vi "Fix Fixed-Point Configuration on Representation Change.vi"(8 "error in (no error)":errorcluster, 11 "Numeric Data Type in":refnum<class "Numeric Data Type.lvclass">) -> (0 "error out":errorcluster, 3 "Numeric Data Type out":refnum<class "Numeric Data Type.lvclass">)   [LabVIEW 2018, in "Numeric Data Type.lvclass"]
uses:
  Numeric Data Type.lvclass
  Fixed-Point Value.ctl
  Numeric Data Type.lvclass/Numeric Data Type.ctl
  <vilib>/fxp/FXPxcontrol/FXP.xctl
  Reference Fixed-Point Configuration.vi
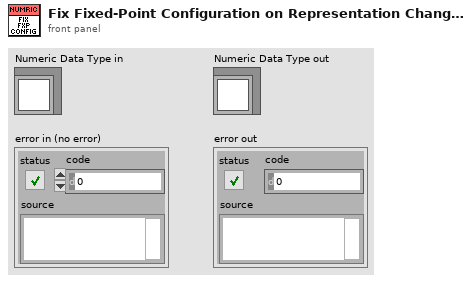
[diagram p1: front panel]
types:
  T1 = typedef "Numeric Data Type.lvclass/Fixed-Point Value.ctl" = cluster{"Encoding":cluster{"Signed":bool, "Word Length":u32, "Integer Word Length":i32}, "Range":cluster{"Range Min":dbl, "Range Max":dbl, "Delta":dbl}}
  T2 = typedef "Numeric Data Type.lvclass/Representation Enum.ctl" = enum16{"Extended (EXT)", "Double (DBL)", "Single (SGL)", "Fixed-Point (FXP)", "Quad Integer (I64)", "Long Integer (I32)", "Word Integer (I16)", "Byte Integer (I8)", "Unsigned Quad (U64)", "Unsigned Long (U32)", "Unsigned Word (U16)", "Unsigned Byte (U8)", "Complex Extended (CXT)", "Complex Double (CDB)", "Complex Single (CSG)"}
  T3 = enum8{"Enabled", "Disabled", "Disabled and Grayed Out"}
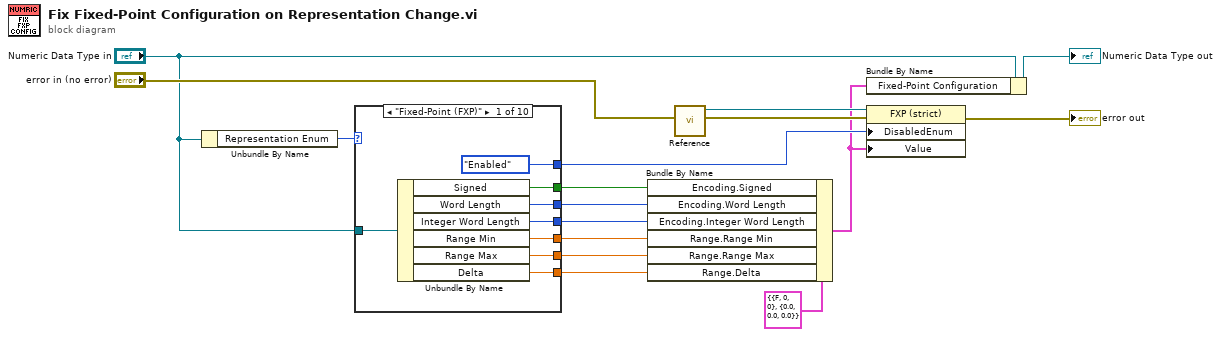
[diagram p0: block diagram]
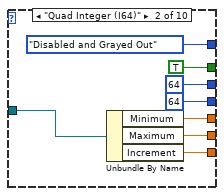
[diagram p2: hidden frame]
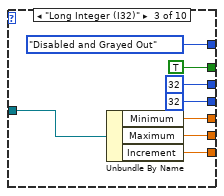
[diagram p3: hidden frame]
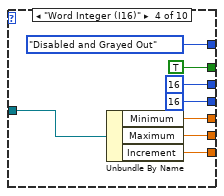
[diagram p4: hidden frame]
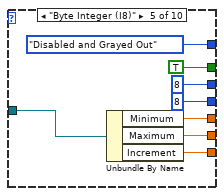
[diagram p5: hidden frame]
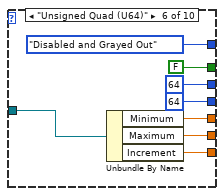
[diagram p6: hidden frame]
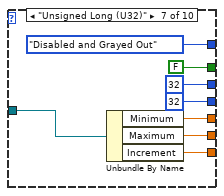
[diagram p7: hidden frame]
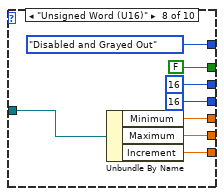
[diagram p8: hidden frame]
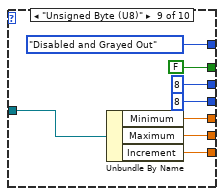
[diagram p9: hidden frame]
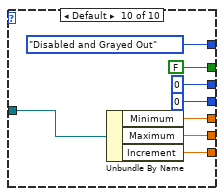
[diagram p10: hidden frame]
diagram:
  n1 = Unbundle By Name("Numeric Data Type in") -> ("Representation Enum"=w14:T2)
  n2 = case shown="\"Fixed-Point (FXP)\"" w14 {
    tunnel: [T3."Enabled" ("Disabled") T3."Disabled and Grayed Out" ("Disabled") T3."Disabled and Grayed Out" ("Disabled") T3."Disabled and Grayed Out" ("Disabled") T3."Disabled and Grayed Out" ("Disabled") T3."Disabled and Grayed Out" ("Disabled") T3."Disabled and Grayed Out" ("Disabled") T3."Disabled and Grayed Out" ("Disabled") T3."Disabled and Grayed Out" ("Disabled") T3."Disabled and Grayed Out" ("Disabled")] -> w7
    tunnel: "Numeric Data Type in" -> [w17 w28 w36 w44 w52 w60 w68 w76 w84 w92]
    tunnel: [w23 TRUE TRUE TRUE TRUE FALSE FALSE FALSE FALSE FALSE] -> w8
    tunnel: [w22 u32 64 u32 32 u32 16 u32 8 u32 64 u32 32 u32 16 u32 8 u32 0] -> w9
    tunnel: [w21 64 32 16 8 64 32 16 8 0] -> w10
    tunnel: [w20 w27 w35 w43 w51 w59 w67 w75 w83 w91] -> w11
    tunnel: [w19 w26 w34 w42 w50 w58 w66 w74 w82 w90] -> w12
    tunnel: [w18 w25 w33 w41 w49 w57 w65 w73 w81 w89] -> w13
    frame "Fixed-Point (FXP)" {
      n3 = Unbundle By Name(w17) -> ("Signed"=w23:bool, "Word Length"=w22:u32, "Integer Word Length"=w21:i32, "Range Min"=w20:dbl, "Range Max"=w19:dbl, "Delta"=w18:dbl)
    }
    frame "Quad Integer (I64)" {
      n4 = Unbundle By Name(w28) -> ("Minimum"=w27:dbl, "Maximum"=w26:dbl, "Increment"=w25:dbl)
    }
    frame "Long Integer (I32)" {
      n5 = Unbundle By Name(w36) -> ("Minimum"=w35:dbl, "Maximum"=w34:dbl, "Increment"=w33:dbl)
    }
    frame "Word Integer (I16)" {
      n6 = Unbundle By Name(w44) -> ("Minimum"=w43:dbl, "Maximum"=w42:dbl, "Increment"=w41:dbl)
    }
    frame "Byte Integer (I8)" {
      n7 = Unbundle By Name(w52) -> ("Minimum"=w51:dbl, "Maximum"=w50:dbl, "Increment"=w49:dbl)
    }
    frame "Unsigned Quad (U64)" {
      n8 = Unbundle By Name(w60) -> ("Minimum"=w59:dbl, "Maximum"=w58:dbl, "Increment"=w57:dbl)
    }
    frame "Unsigned Long (U32)" {
      n9 = Unbundle By Name(w68) -> ("Minimum"=w67:dbl, "Maximum"=w66:dbl, "Increment"=w65:dbl)
    }
    frame "Unsigned Word (U16)" {
      n10 = Unbundle By Name(w76) -> ("Minimum"=w75:dbl, "Maximum"=w74:dbl, "Increment"=w73:dbl)
    }
    frame "Unsigned Byte (U8)" {
      n11 = Unbundle By Name(w84) -> ("Minimum"=w83:dbl, "Maximum"=w82:dbl, "Increment"=w81:dbl)
    }
    frame Default {
      n12 = Unbundle By Name(w92) -> ("Minimum"=w91:dbl, "Maximum"=w90:dbl, "Increment"=w89:dbl)
    }
  }
  n13 = Bundle By Name(cluster=T1 {"Encoding"={"Signed"=FALSE, "Word Length"=0, "Integer Word Length"=0}, "Range"={"Range Min"=0.0, "Range Max"=0.0, "Delta"=0.0}} ("Fixed-Point Configuration"), "Encoding.Signed"=w8, "Encoding.Word Length"=w9, "Encoding.Integer Word Length"=w10, "Range.Range Min"=w11, "Range.Range Max"=w12, "Range.Delta"=w13) -> (w3:T1)
  n14 = call-poly "Reference.vi"("error in (no error)"="error in (no error)") -> ("error out"=w5:errorcluster, "Fixed-Point Configuration"=w4:refnum<vi>)  [unwired: 9 in]
  n15 = Bundle By Name(cluster="Numeric Data Type in", "Fixed-Point Configuration"=w3) -> (→"Numeric Data Type out":refnum<class "Numeric Data Type.lvclass">)
  n16 = property class="FXP (strict)"(reference=w4, error in=w5, "DisabledEnum"=w7, "Value"=w3) -> (error out=→"error out":errorcluster)  [unwired: 1 out]
